vi "GetPulsesFromDvrElement.vi"(9 "length":i32, 10 "index":i32, 11 "DVR element in":T1) -> (1 "count":i32, 2 "pulses":dbl[](array[numeric]))   [LabVIEW 2017, in "DataAccumulator.lvlib"]
uses:
  <vilib>/addons/InsightCM/Devices/Shared/Common/DataAccumulator/DataAccumulator.lvlib
  <vilib>/addons/InsightCM/Devices/Shared/Common/DVRBuffer/controls/DVRElement.ctl
  <vilib>/addons/InsightCM/Devices/Shared/Common/DVRBuffer/DVRBuffer.lvlib
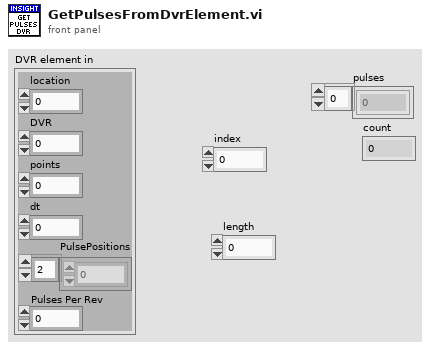
[diagram p1: front panel]
types:
  T1 = typedef "DVRBuffer.lvlib/DVRElement.ctl" = cluster{"location":u32, "DVR":u32, "points":i32, "dt":dbl, "PulsePositions":dbl[], "Pulses Per Rev":dbl}
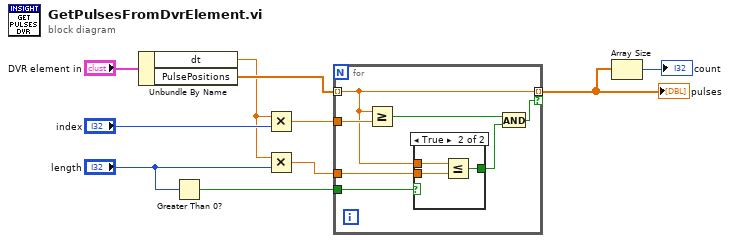
[diagram p0: block diagram]
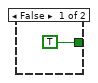
[diagram p2: hidden frame]
diagram:
  n1 = Unbundle By Name("DVR element in") -> ("dt"=w5:dbl, "PulsePositions"=w6:dbl[])
  n2 = Greater Than 0?(x="length") -> (x > 0?=w3:bool)
  n3 = Multiply(x=w5, y="index") -> (x*y=w8:dbl)
  n4 = Multiply(x=w5, y="length") -> (x*y=w2:dbl)
  n5 = for {
    tunnel: w6 -> [w15] mode=indexing
    tunnel: [w15] -> w7 mode=indexing if=w11
    tunnel: w8 -> [w17]
    tunnel: w3 -> [w16]
    tunnel: w2 -> [w14]
    n6 = Greater Or Equal?(x=w15, y=w17) -> (x >= y?=w12:bool)
    n7 = case shown="True" w16 {
      tunnel: w15 -> [_ w21]
      tunnel: w14 -> [_ w20]
      tunnel: [TRUE w19] -> w13
      frame False {
      }
      frame True {
        n8 = Less Or Equal?(x=w21, y=w20) -> (x <= y?=w19:bool)
      }
    }
    n9 = And(x=w12, y=w13) -> (x .and. y?=w11:bool)
  }
  "pulses" <- w7
  n10 = Array Size(array=w7) -> (size(s)=→"count":i32)
